vi "MeasuringDevice.UnInit.vi"(8 "error in (no error)":errorcluster, 11 "OPM.ThorlabsPM400":refnum<class "OPM.ThorlabsPM400.lvclass">) -> (0 "error out":errorcluster, 3 "OPM.ThorlabsPM400 out":refnum<class "OPM.ThorlabsPM400.lvclass">)   [LabVIEW 2017, in "OPM.ThorlabsPM400.lvclass"]
doc: "---------------------------------------------------------------\nJKI State Machine Objects™\nhttp://jki.net/state-machine-objects/\nCopyright (C) 2005-2015, JKI <info@jki.net>\nALL RIGHTS RESERVEDJKI State Machine Objects (SMO) 1.0.0.5\nJKI - JKI\nCopyright (c) 2016, JKI"
uses:
  OPM.ThorlabsPM400.lvclass
  OPM/OPM.lvclass
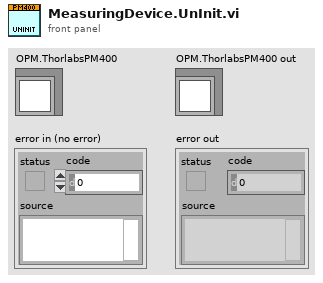
[diagram p1: front panel]
types:
  T1 = typedef "OPM.ThorlabsPM400.lvclass/Resource--Cluster.ctl" = cluster{"Instrument handle":refnum<visa-resource-name>}
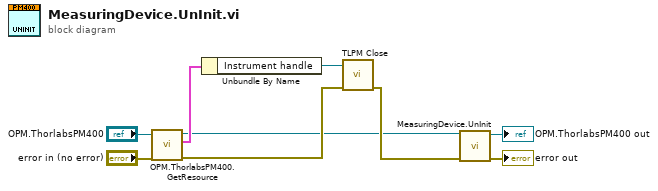
[diagram p0: block diagram]
diagram:
  n1 = call "OPM.ThorlabsPM400.GetResource.vi"("error in (no error)"="error in (no error)", "OPM.ThorlabsPM400 in"="OPM.ThorlabsPM400") -> ("error out"=w3:errorcluster, "Resource"=w5:T1, "OPM.ThorlabsPM400 out"=w1:refnum<class "OPM.ThorlabsPM400.lvclass">)  [unwired: 7 in]
  n2 = Unbundle By Name(w5) -> ("Instrument handle"=w4:refnum<visa-resource-name>)
  n3 = call <instrlib>:"TLPM Close.vi"("error in (no error)"=w3, "instrument handle"=w4) -> ("error out"=w2:errorcluster)  [unwired: 9 in]
  n4 = call-parent "MeasuringDevice.UnInit.vi"("error in (no error)"=w2, "MeasuringDevice"=w1) -> ("error out"=→"error out":errorcluster, "MeasuringDevice out"=→"OPM.ThorlabsPM400 out":refnum<class "OPM.ThorlabsPM400.lvclass">)  [unwired: 8 in]
